vi "Actor Core.vi"(8 "error in":errorcluster, 11 "Universal Display in":refnum<class "Universal Display.lvclass">) -> (0 "error out":errorcluster, 3 "Actor out":refnum<class "Actor.lvclass">)   [LabVIEW 2014, in "Display Panel.lvlib" / "Universal Display.lvclass"]
doc: "(<B>Filename</B>: Actor Framework.lvlib:Actor.lvclass:Actor Core.vi)\n\nReceives messages to the actor, reacts to them, and initiates any error handling that may shut the actor down.\n\nDescendant classes may override this VI to append parallel tasks for the actor to complete while it handles messages. Overrides use the Call Parent Method node."
uses:
  Universal Display.lvclass
  <vilib>/ActorFramework/Actor/Actor.lvclass
  Abstract Display/State.ctl
  Universal Power Meter/Universal Power Meter class/Models.ctl
  Abstract Display/Abstract Display.lvclass/Abstract Display.ctl
  Universal Display.lvclass/Universal Display.ctl
  <vilib>/ActorFramework/Actor/Actor.lvclass/Actor.ctl
  <vilib>/ActorFramework/Message Enqueuer/Message Enqueuer.lvclass/Message Enqueuer.ctl
  Generic Instrument/Generic Card Messages/Write State refnum from Value Msg/Write State refnum from Value Msg.lvclass/Write State refnum from Value Msg.ctl
  <vilib>/ActorFramework/Message Enqueuer/Message Priority.ctl
  Universal Power Meter/Universal Power Meter Messages/Integrator Start-Stop Msg/Integrator Start-Stop Msg.lvclass/Integrator Start-Stop Msg.ctl
  Abstract Display Messages/State Right value from Ref Msg/State Right value from Ref Msg.lvclass/State Right value from Ref Msg.ctl
  <vilib>/ActorFramework/Message Enqueuer/Enqueue.vi
  <vilib>/ActorFramework/Message Enqueuer/Init from Existing Queue.vi
  <vilib>/ActorFramework/Message Priority Queue/Priority Enqueue.vi
  <vilib>/express/express shared/transition.llb/Dynamic To Waveform Array.vi
  <vilib>/express/express signal manip/GetorSetDDTAttributes/Set DDT Attributes/SetT0.vi
  <vilib>/express/express shared/transition.llb/Waveform Array To Dynamic.vi
  <vilib>/ActorFramework/Message Enqueuer/Message Enqueuer.lvclass
  Generic Instrument/Generic Card Messages/Write State refnum from Value Msg/Write State refnum from Value Msg.lvclass
  <vilib>/express/express signal manip/GetorSetDDTAttributes/Set DDT Attributes/Set DDT Properties.xnode
  <vilib>/ActorFramework/Stop Msg/Stop Msg.lvclass
  Universal Power Meter/Universal Power Meter Messages/Integrator Start-Stop Msg/Integrator Start-Stop Msg.lvclass
  <vilib>/express/express signal manip/GetorSetDDTAttributes/Get DDT Attributes/Get DDT Properties.xnode
  Abstract Display Messages/State Right value from Ref Msg/State Right value from Ref Msg.lvclass
  Abstract Display/Abstract Display.lvclass
  Data Logger/Data Logger.lvclass
panel:
  out "Elapsed Time (s)":dbl
  out "number of logs":i32
  out "logger i":i32
  out "Current State":T1
  out "i":i32
  in  "Measurement Interval":dbl
  out "Instrument Name":string
  out "Address to save":string
  in  "Waveform Chart":dynamicdata(graph)
  in  "Cluster":T2
  out "Array 2":T3(array[cluster])
  out "Card #":dbl
  in  "Exit":bool
  out "Time":dbl format="%<%H:%M:%S>t"
  out "Blinker":bool
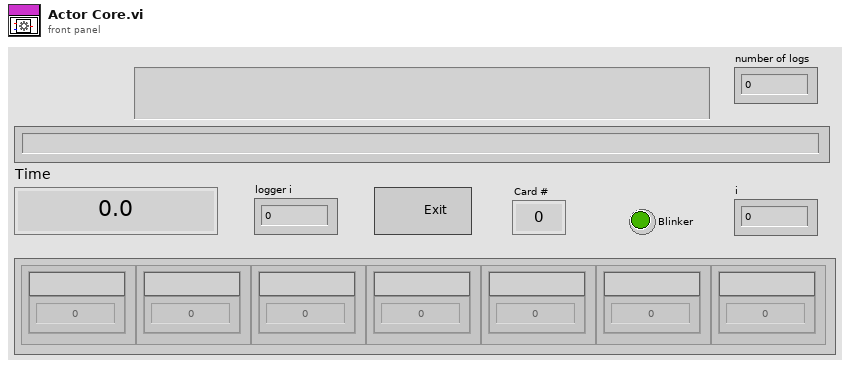
[diagram p1: front panel]
types:
  T1 = typedef "Display Panel.lvlib/Abstract Display.lvclass/State.ctl" = enum16{"Done", "Warming", "Measuring"}
  T2 = cluster{"Numeric Indicator 2":dbl, "String":string}
  T3 = cluster{"Numeric Indicator 2":dbl, "String":string}[]
  T4 = typedef "Models.ctl" = enum16{"PA1000", "USB-6501", "2635A", "2625A", "WT500", "WT1600", "DMM4020", "WT230", "WT210"}
  T5 = typedef "Actor Framework.lvlib/Message Enqueuer.lvclass/Message Priority.ctl" = enum16{"Low", "Normal", "High"}
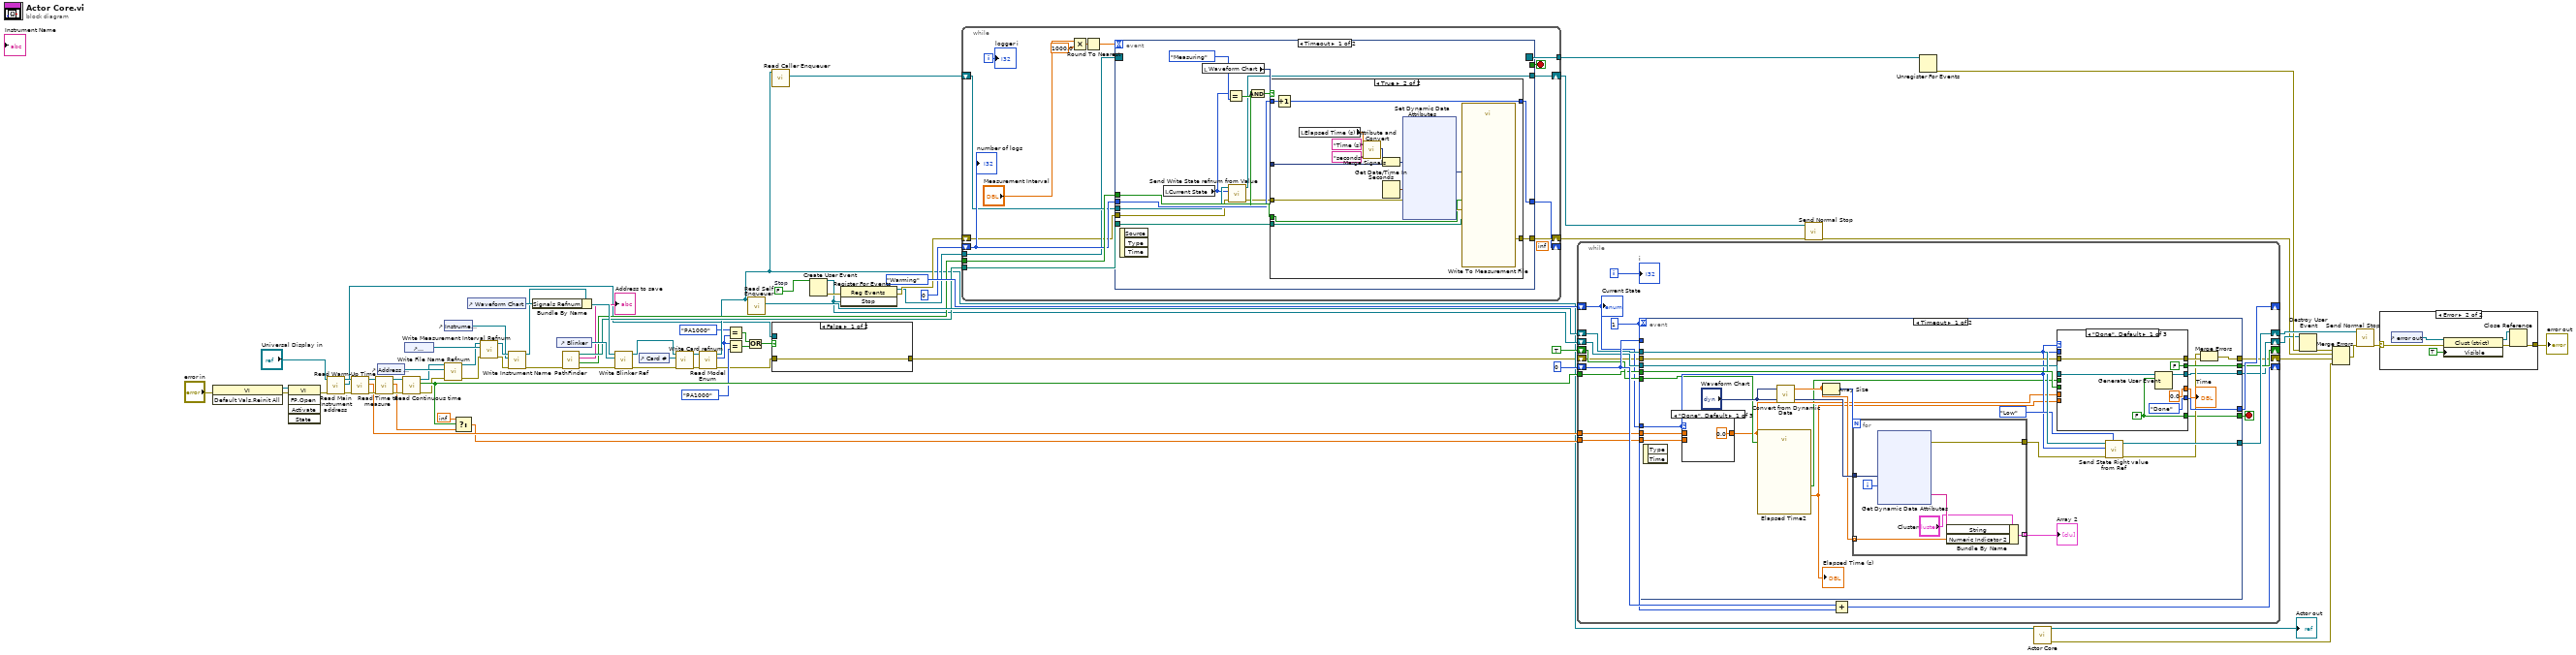
[diagram p0: block diagram]
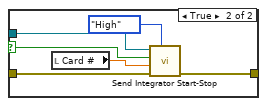
[diagram p2: hidden frame]
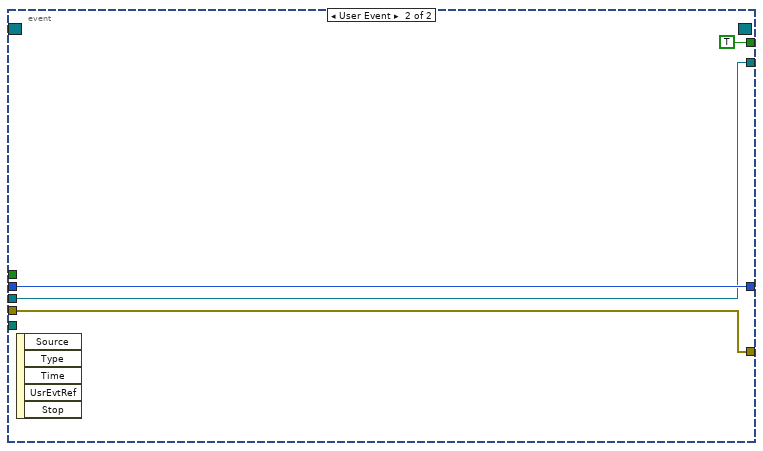
[diagram p4: hidden frame]
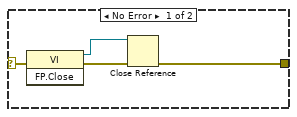
[diagram p5: hidden frame]
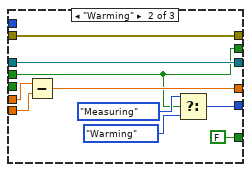
[diagram p8: hidden frame]
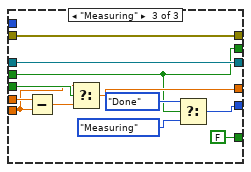
[diagram p9: hidden frame]
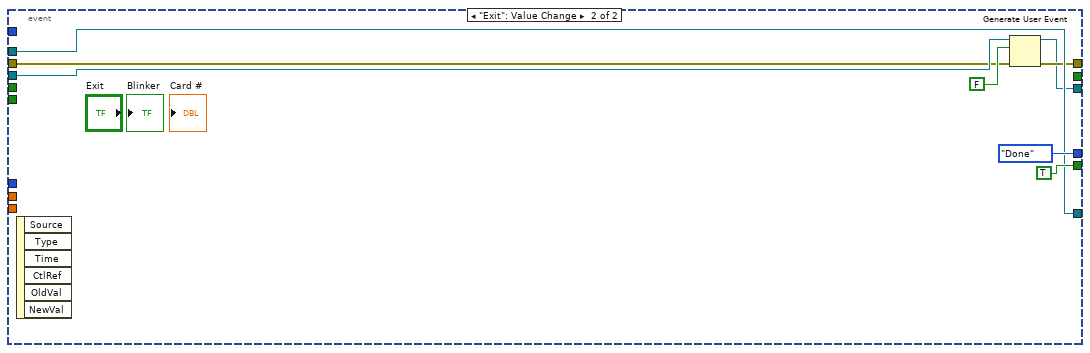
[diagram p10: hidden frame]
diagram:
  w29 = FALSE  # Stop
  n1 = invoke class="VI" method="Default Vals.Reinit All"(error in="error in") -> (reference out=w73:refnum<vi>, error out=w67:errorcluster)  [unwired: 2 in, 1 out]
  n2 = invoke class="VI" method="FP.Open"(reference=w73, error in=w67) -> (error out=w6:errorcluster)  [unwired: 3 in, 4 out]
  n3 = call-dynamic "Read Main Instrument address.vi"("error in (no error)"=w6, "Abstract Display in"="Universal Display in") -> ("error out"=w5:errorcluster, "Actor Framework:Message Enqueuer"=w3:refnum<class "Message Enqueuer.lvclass">, "Abstract Display out"=w4:refnum<class "Universal Display.lvclass">)  [unwired: 7 in]
  n4 = call-dynamic "Read Warm-Up Time.vi"("error in (no error)"=w5, "Abstract Display in"=w4) -> ("error out"=w58:errorcluster, "Warm-Up Time"=w51:dbl, "Abstract Display out"=w59:refnum<class "Universal Display.lvclass">)  [unwired: 7 in]
  n5 = call-dynamic "Read Time to measure.vi"("error in (no error)"=w58, "Abstract Display in"=w59) -> ("error out"=w56:errorcluster, "Time to measure"=w54:dbl, "Abstract Display out"=w57:refnum<class "Universal Display.lvclass">)  [unwired: 7 in]
  n6 = control-ref of="Address to save"() -> (w64:refnum<vi>)
  n7 = call-dynamic "Read Continuous time.vi"("error in (no error)"=w56, "Abstract Display in"=w57) -> ("error out"=w44:errorcluster, "Continuous time"=w45:bool, "Abstract Display out"=w55:refnum<class "Universal Display.lvclass">)  [unwired: 7 in]
  n8 = control-ref of="Measurement Interval"() -> (w49:refnum<vi>)
  n9 = control-ref of="Instrument Name"() -> (w60:refnum<vi>)
  n10 = call "Write File Name Refnum.vi"("error in (no error)"=w44, "File Name Refnum"=w64, "Abstract Display in"=w55) -> ("error out"=w63:errorcluster, "Abstract Display out"=w18:refnum<class "Universal Display.lvclass">)  [unwired: 7 in]
  n11 = Select(t=inf, s=w45, f=w54) -> (s? t:f=w50:dbl)
  n12 = control-ref of="Waveform Chart"() -> (w68:refnum<vi>)
  n13 = call "Write Measurement Interval Refnum.vi"("error in (no error)"=w63, "Measurement Interval Refnum"=w49, "Abstract Display in"=w18) -> ("error out"=w62:errorcluster, "Abstract Display out"=w61:refnum<class "Universal Display.lvclass">)  [unwired: 7 in]
  n14 = call "Write Instrument Name.vi"("error in (no error)"=w62, "Instrument Name"=w60, "Abstract Display in"=w61) -> ("error out"=w39:errorcluster, "Abstract Display out"=w17:refnum<class "Universal Display.lvclass">)  [unwired: 7 in]
  n15 = Bundle By Name(cluster=w17, "Signals Refnum"=w68) -> (w69:refnum<class "Universal Display.lvclass">)
  n16 = control-ref of="Blinker"() -> (w72:refnum<vi>)
  n17 = call "PathFinder.vi"("error in"=w39) -> ("error out"=w36:errorcluster, "Save?"=w37:bool, "Path"=→"Address to save":string, "selected path"=w38:path)  [unwired: 7 in]
  n18 = call "Write Blinker Ref.vi"("error in (no error)"=w36, "Blinker Ref"=w72, "Abstract Display in"=w69) -> ("error out"=w46:errorcluster, "Abstract Display out"=w47:refnum<class "Universal Display.lvclass">)  [unwired: 7 in]
  n19 = control-ref of="Card #"() -> (w70:refnum<vi>)
  n20 = call "Write Card refnum.vi"("error in (no error)"=w46, "Card refnum"=w70, "Abstract Display in"=w47) -> ("error out"=w15:errorcluster, "Abstract Display out"=w16:refnum<class "Universal Display.lvclass">)  [unwired: 7 in]
  n21 = call-dynamic "Read Model Enum.vi"("error in (no error)"=w15, "Abstract Display in"=w16) -> ("error out"=w2:errorcluster, "Enum"=w11:T4, "Abstract Display out"=w14:refnum<class "Universal Display.lvclass">)  [unwired: 7 in]
  n22 = Equal?(x=Models."PA1000" ("Enum"), y=w11) -> (x = y?=w13:bool)
  n23 = Equal?(x=w11, y=Models."PA1000" ("Enum")) -> (x = y?=w12:bool)
  n24 = Or(x=w13, y=w12) -> (x .or. y?=w8:bool)
  n25 = call <vilib>:"Read Self Enqueuer.vi"("Actor"=w14) -> ("Self Enqueuer"=w40:refnum<class "Message Enqueuer.lvclass">)  [unwired: 10 in]
  n26 = call <vilib>:"Read Caller Enqueuer.vi"("Actor"=w14) -> ("Caller Enqueuer"=w33:refnum<class "Message Enqueuer.lvclass">)  [unwired: 10 in]
  n27 = case shown="False" w8 {
    selector: w8 -> [_ w81]
    tunnel: w3 -> [_ w80]
    tunnel: w2 -> [w75 w78]
    tunnel: [w75 w77] -> w1
    frame False {
    }
    frame True {
      n28 = local read "Card #"() -> (w79:dbl)
      n29 = call "Send Integrator Start-Stop.vi"("Message Priority (Normal)"=Message_Priority."High", "error in (no error)"=w78, "Element (All: 0)"=w79, "Start/Stop (F: Stop)"=w81, "Message Enqueuer"=w80) -> ("error out"=w77:errorcluster)  [unwired: 5 in, 1 out]
    }
  }
  n30 = Create User Event(user event datatype=w29) -> (user event=w24:refnum<user-event>, error out=w28:errorcluster)  [unwired: 1 in]
  n31 = register-events(error in=w28, w24) -> (reference out=w26:refnum<event-registration>, error out=w27:errorcluster)  [unwired: 1 in]
  n32 = while {
    tunnel: w38 -> [w97]
    tunnel: w37 -> [w96]
    shift-right: [w95] -> w31
    shift-left: w27 -> [w82]
    shift-right: [w87] -> _
    shift-left: 0 -> [w88]
    shift-right: [w85] -> w32
    shift-left: w33 -> [w86]
    tunnel: w26 -> [w84]
    tunnel: [w83] -> w25
    i -> [w89]
    stop <- w90 stop-if-true
    (unwired) inf
    n33 = Multiply(x="Measurement Interval", y=1000.0) -> (x*y=w92:dbl)
    n34 = Round To Nearest(number=w92) -> (nearest integer value=w91:dbl)
    n35 = event shown="[0] Timeout" {
      selector: w84 -> [_ _]
      dyn-events: [_ _] -> w83
      timeout: w91 -> [_ _]
      tunnel: w97 -> [w110 _]
      tunnel: w96 -> [w108 _]
      tunnel: w82 -> [w100 w143]
      tunnel: [w109 w143] -> w95
      tunnel: [_ TRUE] -> w90
      tunnel: w88 -> [w104 w145]
      tunnel: [w103 w145] -> w87
      tunnel: w86 -> [w102 w144]
      tunnel: [w98 w144] -> w85
      event Timeout {
        n36 = event-data() -> ()  [unwired: 1 in, 3 out]
        n37 = local read "Current State"() -> (w99:T1)
        n38 = local read "Waveform Chart"() -> (w111:dynamicdata)
        n39 = Equal?(x=w99, y=State."Measuring" ("States")) -> (x = y?=w106:bool)
        n40 = call "Send Write State refnum from Value.vi"("error in (no error)"=w100, "States"=w99, "Message Enqueuer"=w102) -> ("error out"=w101:errorcluster, "Message Enqueuer out"=w98:refnum<class "Message Enqueuer.lvclass">)  [unwired: 7 in]
        n41 = And(x=w108, y=w106) -> (x .and. y?=w105:bool)
        n42 = case shown="True" w105 {
          tunnel: w101 -> [w113 w117]
          tunnel: w111 -> [_ w125]
          tunnel: [w113 w118] -> w109
          tunnel: w108 -> [_ w121]
          tunnel: w110 -> [_ w120]
          tunnel: w104 -> [w112 w116]
          tunnel: [w112 w115] -> w103
          frame False {
          }
          frame True {
            n43 = Increment(x=w116) -> (x+1=w115:i32)
            n44 = local read "Elapsed Time (s)"() -> (w114:dbl)
            n45 = call "Attribute and Convert.vi"("Unit"="seconds", "Signal Name"="Time (s)", "Number in"=w114) -> ("Dynamic Signal Out"=w127:dynamicdata)  [unwired: 8 in]
            n46 = Merge Signals(w127, w125) -> (w119:dynamicdata)
            n47 = Get Date/Time In Seconds() -> (seconds since 1Jan1904=w123:timestamp)
            n48 = xnode "Set Dynamic Data Attributes"("Signals In"=w119, "Timestamp"=w123, "error in"=w117) -> ("Signals Out"=w122:dynamicdata, "error out"=w124:errorcluster)  [unwired: 1 in]
            n49 = call "Write To Measurement File"("Signals"=w122, "Enable"=w121, "error in (no error)"=w124, "Filename"=w120) -> ("error out"=w118:errorcluster)  [unwired: 13 in, 2 out]
          }
        }
      }
      event User Event {
        n50 = event-data() -> ()  [unwired: 1 in, 5 out]
      }
    }
    "logger i" <- w89
    "number of logs" <- w88
  }
  n51 = while {
    shift-right: [w163] -> _
    shift-left: 0 -> [w164]
    tunnel: w51 -> [w162]
    tunnel: w50 -> [w161]
    shift-right: [w160] -> _
    shift-left: State."Warming" ("States") -> [w150]
    shift-right: [w158] -> w41
    shift-left: w40 -> [w159]
    shift-right: [w156] -> _
    shift-left: TRUE ("Open Actor Core front panel? (F)") -> [w157]
    tunnel: w45 -> [w155]
    shift-right: [w148] -> w23
    shift-left: w24 -> [w151]
    shift-right: [w147] -> w20
    shift-left: w1 -> [w149]
    i -> [w154]
    stop <- w153 stop-if-true
    w152 = 1
    n52 = event shown="[0] Timeout" {
      selector: _ -> [_ _]
      dyn-events: _ -> [_ _]
      timeout: w152 -> [_ _]
      tunnel: w164 -> [_ _]
      tunnel: [w176 TRUE] -> w153
      tunnel: [w177 w242] -> w147
      tunnel: w149 -> [w175 w240]
      tunnel: w150 -> [w171 _]
      tunnel: w162 -> [w169 _]
      tunnel: w161 -> [w168 _]
      tunnel: [w189 State."Done" ("States")] -> w160
      tunnel: w159 -> [w183 w244]
      tunnel: [w182 w244] -> w158
      tunnel: w157 -> [w170 _]
      tunnel: [w188 _] -> w156
      tunnel: w155 -> [w187 _]
      tunnel: w151 -> [w172 w243]
      tunnel: [w173 w239] -> w148
      event Timeout {
        n53 = event-data() -> ()  [unwired: 1 in, 2 out]
        n54 = case shown="\"Done\", Default" w171 {
          tunnel: w169 -> [_ w192 _]
          tunnel: [0.0 ("Time to measure") w192 w193] -> w167
          tunnel: w168 -> [_ _ w193]
          frame "Done", Default {
          }
          frame "Warming" {
          }
          frame "Measuring" {
          }
        }
        n55 = call "Elapsed Time2"("Time Target (s)"=w167, "Reset"=w170) -> ("Elapsed Time (s)"=w166:dbl, "Time has Elapsed"=w165:bool)  [unwired: 10 in, 6 out]
        "Elapsed Time (s)" <- w166
        n56 = call "Convert from Dynamic Data"("Dynamic Data Type"="Waveform Chart") -> ("Array"=w181:dbl[])  [unwired: 3 in]
        n57 = Array Size(array=w181) -> (size(s)=w185:i32)
        n58 = for {
          N: w185 -> [_]
          tunnel: "Waveform Chart" -> [w229]
          tunnel: [w227] -> w190 mode=indexing
          tunnel: [w224] -> w179
          tunnel: w181 -> [w223] mode=indexing
          i -> [w228]
          n59 = xnode "Get Dynamic Data Attributes"("Signals In"=w229, "Signal Index"=w228) -> ("Signal Name"=w226:string, "error out"=w224:errorcluster)  [unwired: 1 in, 1 out]
          n60 = Bundle By Name(cluster="Cluster", "String"=w226, "Numeric Indicator 2"=w223) -> (w227:T2)
        }
        "Array 2" <- w190
        n61 = case shown="\"Done\", Default" w171 {
          tunnel: w171 -> [_ _ _]
          tunnel: [State."Done" ("States") w210 w217] -> w189
          tunnel: [FALSE ("Time has Elapsed") w202 w211] -> w188
          tunnel: w187 -> [_ _ w222]
          tunnel: w175 -> [w197 w201 w212]
          tunnel: [0.0 ("Elapsed Time (s)") w209 w220] -> w186
          tunnel: [w197 w201 w212] -> w180
          tunnel: [w196 FALSE FALSE] -> w176
          tunnel: [w195 w205 w215] -> w173
          tunnel: w172 -> [w194 w205 w215]
          tunnel: w167 -> [_ w204 w214]
          tunnel: w166 -> [_ w203 w213]
          tunnel: w165 -> [_ w202 w211]
          frame "Done", Default {
            w196 = FALSE
            n62 = Generate User Event(user event=w194, event data cluster=w196) -> (user event out=w195:refnum<user-event>)  [unwired: 2 in, 1 out]
          }
          frame "Warming" {
            n63 = Subtract(x=w204, y=w203) -> (x-y=w209:dbl)
            n64 = Select(t=State."Measuring" ("States"), s=w202, f=State."Warming" ("States")) -> (s? t:f=w210:T1)
          }
          frame "Measuring" {
            n65 = Subtract(x=w214, y=w213) -> (x-y=w221:dbl)
            n66 = Select(t=w213, s=w222, f=w221) -> (s? t:f=w220:dbl)
            n67 = Select(t=State."Done" ("States"), s=w211, f=State."Measuring" ("States")) -> (s? t:f=w217:T1)
          }
        }
        "Time" <- w186
        n68 = call "Send State Right value from Ref.vi"("Message Priority (Normal)"=Message_Priority."Low", "error in (no error)"=w179, "States"=w171, "Message Enqueuer"=w183) -> ("error out"=w178:errorcluster, "Message Enqueuer out"=w182:refnum<class "Message Enqueuer.lvclass">)  [unwired: 6 in]
        n69 = Merge Errors(w178, w180) -> (w177:errorcluster)
      }
      event "Exit": Value Change {
        n70 = event-data() -> ()  [unwired: 1 in, 6 out]
        n71 = Generate User Event(user event=w243, event data cluster=FALSE ("event data"), error in=w240) -> (user event out=w239:refnum<user-event>, error out=w242:errorcluster)  [unwired: 1 in]
      }
    }
    n72 = Add(x=w164, y=w152) -> (x+y=w163:i32)
    "i" <- w154
    "Current State" <- w150
  }
  n73 = call <vilib>:"Send Normal Stop.vi"("error in (no error)"=w31, "Message Enqueuer"=w32) -> ("error out"=w22:errorcluster)  [unwired: 9 in]
  n74 = Unregister For Events(event registration refnum=w25) -> (error out=w30:errorcluster)  [unwired: 1 in]
  n75 = call-parent "Actor Core.vi"("Abstract Display in"=w14) -> ("error out"=w65:errorcluster, "Actor out"=→"Actor out":refnum<class "Actor.lvclass">)  [unwired: 9 in]
  n76 = Destroy User Event(user event=w23, error in=w30) -> (error out=w19:errorcluster)
  n77 = Merge Errors(w19, w22, w20, w65) -> (w43:errorcluster)
  n78 = call <vilib>:"Send Normal Stop.vi"("error in (no error)"=w43, "Message Enqueuer"=w41) -> ("error out"=w42:errorcluster)  [unwired: 9 in]
  n79 = case shown="Error" w42 {
    selector: w42 -> [w250 w255]
    tunnel: [w247 w251] -> w21
    frame No Error {
      n80 = invoke class="VI" method="FP.Close"(error in=w250) -> (reference out=w248:refnum<vi>, error out=w249:errorcluster)  [unwired: 2 in, 1 out]
      n81 = Close Reference(reference=w248, error in (no error)=w249) -> (error out=w247:errorcluster)
    }
    frame Error {
      n82 = control-ref of="error out"() -> (w256:refnum<vi>)
      n83 = property class="Clust (strict)"(reference=w256, error in=w255, "Visible"=TRUE) -> (reference out=w253:refnum<vi>, error out=w252:errorcluster)
      n84 = Close Reference(reference=w253, error in (no error)=w252) -> (error out=w251:errorcluster)
    }
  }
  "error out" <- w21
